vi "Tacking Helper - Filler Tack Point.vi"(4 "Waypoint Array":T1[](array[typedef]) {"UTM Location"."North" format="%#_10f"; "UTM Location"."East" format="%#_8f"}, 6 "Distance to boat":dbl, 9 "Final Index of Waypoint Array":i32, 10 "Starting Angle":dbl, 11 "Angle from boat to waypoint":dbl) -> (3 "Finalized Waypoint Array":T1[](array[typedef]) {"UTM Location"."North" format="%#_10f"; "UTM Location"."East" format="%#_8f"})   [LabVIEW 2011]
doc: "This vi takes a tack pattern along with the leftover distance to the boat, and extrapolates the angle last used to get the last intermediate waypoint. If done as originally intended, this occurs after all of the jumps, is the only point that doesn't contact the bounding box, and is the closest waypoint to the boat."
uses:
  <vilib>/Analysis/NI_AAL_Angle.lvlib
  <vilib>/Analysis/coordinate.llb/Absolute Angle Difference (scalar).vi
  2 Typedefs/UTM Location.ctl
  0x2-OCU-Think Comm/0x2 Typedefs/ocuWaypoint.ctl
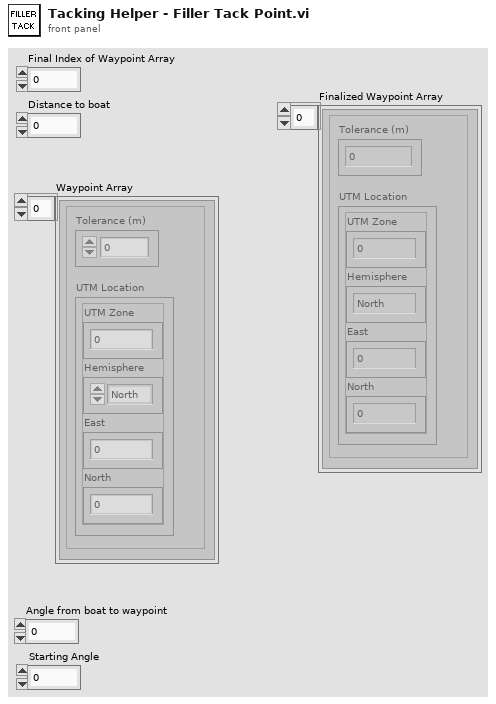
[diagram p1: front panel]
types:
  T1 = typedef "ocuWaypoint.ctl" = cluster{"Tolerance (m)":dbl, "UTM Location":T2}
  T2 = typedef "UTM Location.ctl" = cluster{"UTM Zone":dbl, "Hemisphere":enum16{"North", "South"}, "East":dbl, "North":dbl}
  T3 = typedef "waypointTypes.ctl" = enum16{"Drive", "Round Port", "Round Starboard", "Stay"}
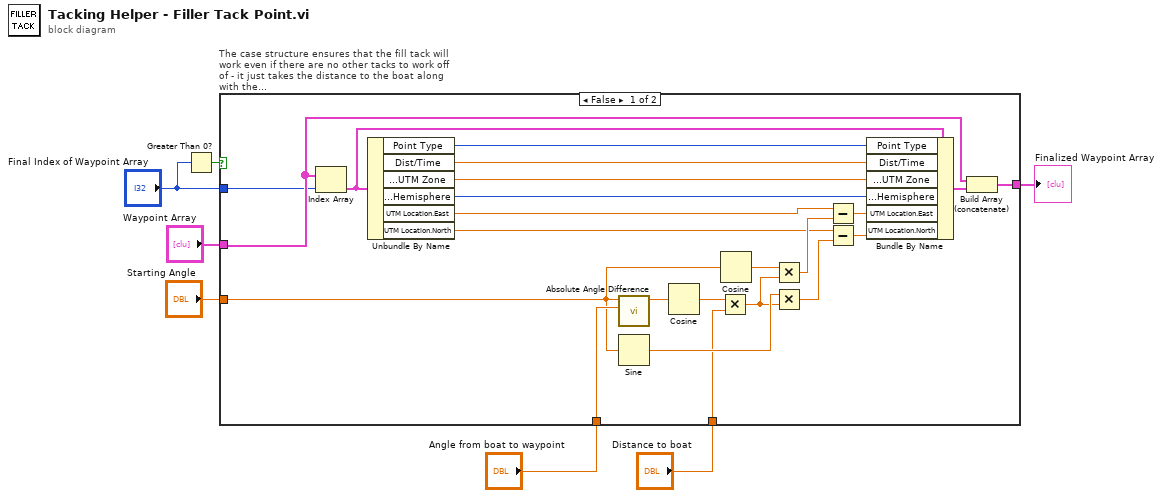
[diagram p0: block diagram]
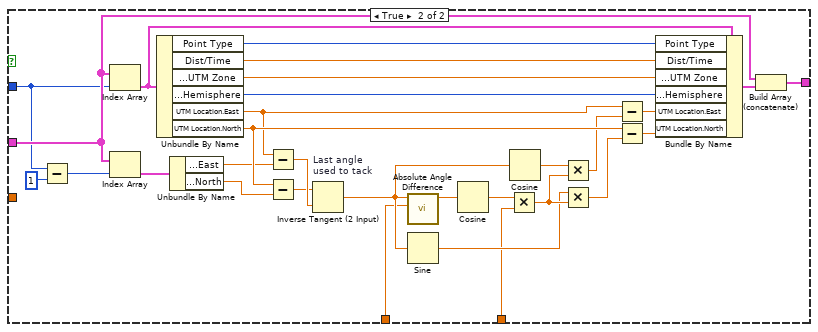
[diagram p2: hidden frame]
diagram:
  n1 = Greater Than 0?(x="Final Index of Waypoint Array") -> (x > 0?=w3:bool)
  n2 = case "The case structure ensures that the fill tack will work even if there are no other tacks to work off of - it just takes the distance to the boat along with the\nstarting angle and fills in the central tack point." shown="False" w3 {
    tunnel: [w9 w47] -> w4
    tunnel: "Waypoint Array" -> [w13 w35]
    tunnel: "Final Index of Waypoint Array" -> [w12 w34]
    tunnel: "Distance to boat" -> [w10 w32]
    tunnel: "Angle from boat to waypoint" -> [w11 w31]
    tunnel: "Starting Angle" -> [w8 _]
    frame False {
      n3 = Index Array(array=w13, index=w12) -> (element=w30:T1)
      n4 = Unbundle By Name(w30) -> ("Point Type"=w28:T3, "Dist/Time"=w27:dbl, "UTM Location.UTM Zone"=w26:dbl, "UTM Location.Hemisphere"=w25:enum16{"North", "South"}, "UTM Location.East"=w15:dbl, "UTM Location.North"=w14:dbl)
      n5 = call-poly <vilib>:"Absolute Angle Difference.vi"("angle 2"=w11, "angle 1"=w8) -> ("absolute angle difference"=w24:dbl)  [unwired: 8 in, 1 out]
      n6 = Sine(x=w8) -> (sin(x)=w21:dbl)
      n7 = Cosine(x=w24) -> (cos(x)=w23:dbl)
      n8 = Multiply(x=w23, y=w10) -> (x*y=w20:dbl)
      n9 = Cosine(x=w8) -> (cos(x)=w22:dbl)
      n10 = Multiply(x=w22, y=w20) -> (x*y=w19:dbl)
      n11 = Multiply(x=w21, y=w20) -> (x*y=w18:dbl)
      n12 = Subtract(x=w15, y=w19) -> (x-y=w17:dbl)
      n13 = Subtract(x=w14, y=w18) -> (x-y=w16:dbl)
      n14 = Bundle By Name(cluster=w30, "Point Type"=w28, "Dist/Time"=w27, "UTM Location.UTM Zone"=w26, "UTM Location.Hemisphere"=w25, "UTM Location.East"=w17, "UTM Location.North"=w16) -> (w29:T1)
      n15 = Build Array (concatenate)(w13, w29) -> (w9:T1[])
    }
    frame True {
      n16 = Subtract(x=w34, y=1) -> (x-y=w43:i32)
      n17 = Index Array(array=w35, index=w34) -> (element=w36:T1)
      n18 = Index Array(array=w35, index=w43) -> (element=w44:T1)
      n19 = Unbundle By Name(w36) -> ("Point Type"=w38:T3, "Dist/Time"=w39:dbl, "UTM Location.UTM Zone"=w40:dbl, "UTM Location.Hemisphere"=w41:enum16{"North", "South"}, "UTM Location.East"=w59:dbl, "UTM Location.North"=w60:dbl)
      n20 = Unbundle By Name(w44) -> ("UTM Location.East"=w58:dbl, "UTM Location.North"=w33:dbl)
      n21 = Subtract(x=w59, y=w58) -> (x-y=w46:dbl)
      n22 = Subtract(x=w60, y=w33) -> (x-y=w45:dbl)
      n23 = Inverse Tangent (2 Input) "Last angle\nused to tack"(1:w46, 2:w45) -> (0:w50:dbl)
      n24 = call-poly <vilib>:"Absolute Angle Difference.vi"("angle 2"=w31, "angle 1"=w50) -> ("absolute angle difference"=w48:dbl)  [unwired: 8 in, 1 out]
      n25 = Sine(x=w50) -> (sin(x)=w52:dbl)
      n26 = Cosine(x=w48) -> (cos(x)=w49:dbl)
      n27 = Multiply(x=w49, y=w32) -> (x*y=w53:dbl)
      n28 = Cosine(x=w50) -> (cos(x)=w51:dbl)
      n29 = Multiply(x=w51, y=w53) -> (x*y=w54:dbl)
      n30 = Multiply(x=w52, y=w53) -> (x*y=w55:dbl)
      n31 = Subtract(x=w59, y=w54) -> (x-y=w56:dbl)
      n32 = Subtract(x=w60, y=w55) -> (x-y=w57:dbl)
      n33 = Bundle By Name(cluster=w36, "Point Type"=w38, "Dist/Time"=w39, "UTM Location.UTM Zone"=w40, "UTM Location.Hemisphere"=w41, "UTM Location.East"=w56, "UTM Location.North"=w57) -> (w37:T1)
      n34 = Build Array (concatenate)(w35, w37) -> (w47:T1[])
    }
  }
  "Finalized Waypoint Array" <- w4
